vi "题目四.vi"() -> ()   [LabVIEW 2017]
uses:
  <vilib>/Utility/file.llb/Write Delimited Spreadsheet (string).vi
  <vilib>/measure/NI_MABase.lvlib
panel:
  out "new file path (Not A Path if cancelled)":path caption="新建文件路径（取消时为非法路径）"
  out "添加的数组":dbl[][](array[numeric])
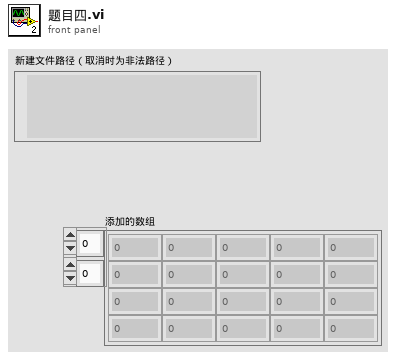
[diagram p1: front panel]
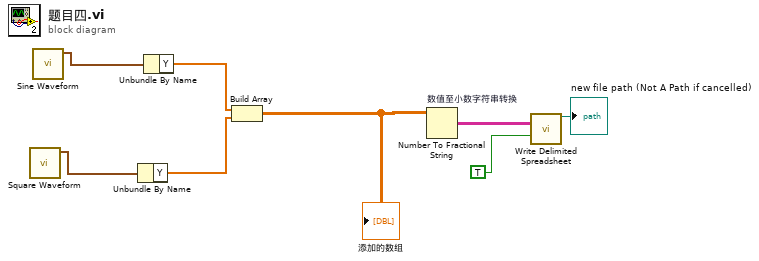
[diagram p0: block diagram]
diagram:
  n1 = call <vilib>:"Square Waveform.vi"() -> ("signal out"=w8:waveform(dbl))  [unwired: 10 in, 1 out]
  n2 = call <vilib>:"Sine Waveform.vi"() -> ("signal out"=w7:waveform(dbl))  [unwired: 10 in, 1 out]
  n3 = Unbundle By Name(w8) -> ("Y"=w5:dbl[])
  n4 = Unbundle By Name(w7) -> ("Y"=w6:dbl[])
  n5 = Build Array(w6, w5) -> (w4:dbl[][])
  "添加的数组" <- w4
  n6 = Number To Fractional String "数值至小数字符串转换"(number=w4) -> (F-format string=w3:string[][])  [unwired: 3 in]
  n7 = call-poly <vilib>:"Write Delimited Spreadsheet.vi"("2D data"=w3, "append to file? (new file:F)"=TRUE) -> ("new file path (Not A Path if cancelled)"=→"new file path (Not A Path if cancelled)":path)  [unwired: 12 in, 1 out]
